vi "Receive Topic Message.vi"(7 "Topic Actor in":refnum<class "Topic Actor.lvclass">, 8 "error in (no error)":errorcluster, 10 "Message in":refnum<class "Message Interface.lvclass">) -> (0 "error out":errorcluster, 3 "Stop?":bool, 5 "Topic Actor out":refnum<class "Topic Actor.lvclass">)   [LabVIEW 2016, in "Stream Mediator.lvlib" / "Topic Actor.lvclass"]
doc: "--\nCopyright © 2017 Composed SystemsI All rights reserved.\n\nAuthor: Jon McBee <jon.mcbee@composed.io>\n\nThis library is provided \"AS IS\" ,WITHOUT WARRANTIES OR\nCONDITIONS OF ANY KIND, either express or implied.\n\nComposed Systems -- composed.io\n\nStream 0.0.1.1\nJon McBee - Composed Systems\nCopyright (c) 2017, Composed Systems"
uses:
  <userlib>/Composed Systems/Stream/Mediator/Classes/Topic Actor/Topic Actor.lvclass
  <userlib>/Composed Systems/Stream/Mediator/Classes/Message Interface/Message Interface.lvclass
  <userlib>/Composed Systems/Stream/Mediator/Classes/Topic Actor Command Interface/Topic Actor Command Interface.lvclass
  <userlib>/Composed Systems/Stream/Mediator/Classes/Topic Actor/Topic Actor.lvclass/Topic Actor.ctl
  <userlib>/Composed Systems/Stream/Mediator/Classes/Message Transport Interface/Message Transport Interface.lvclass
  <userlib>/Composed Systems/Stream/Mediator/Classes/Subscriber Look Up Table/Subscriber Look Up Table.lvclass
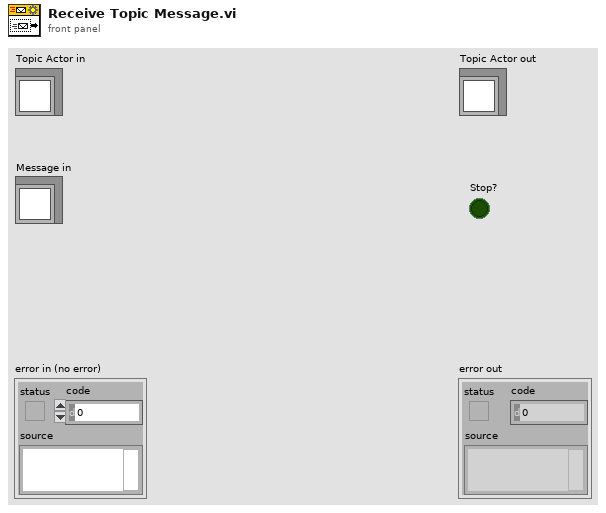
[diagram p1: front panel]
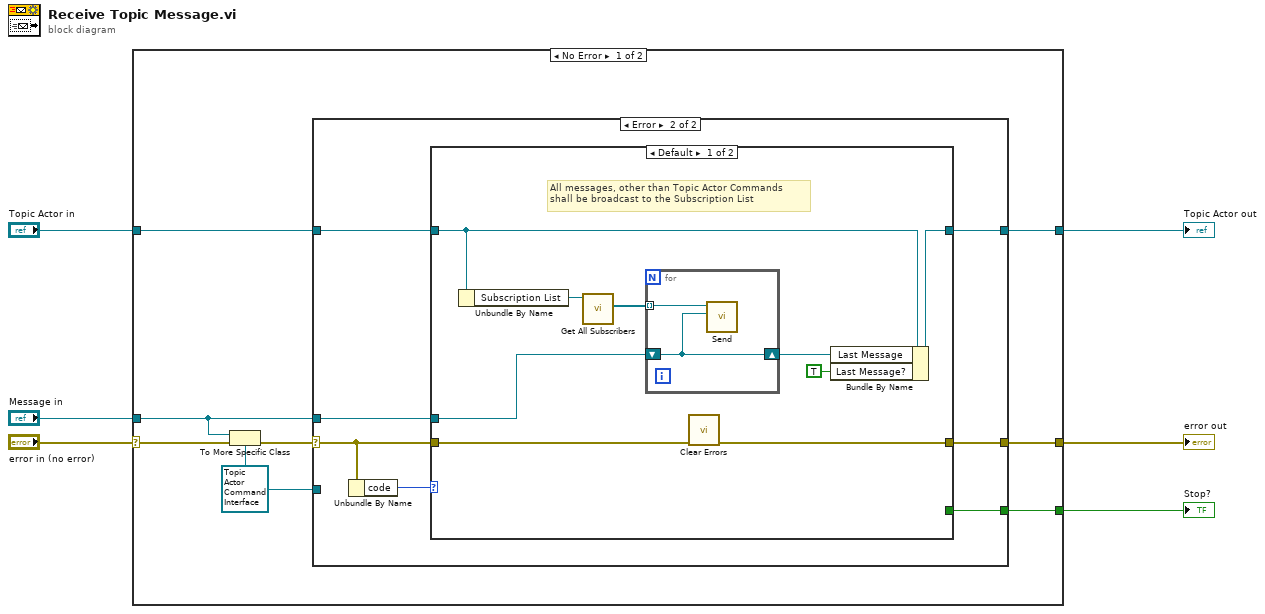
[diagram p0: block diagram]
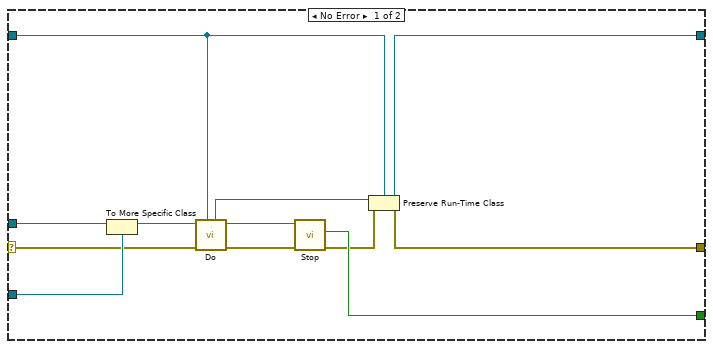
[diagram p2: hidden frame]
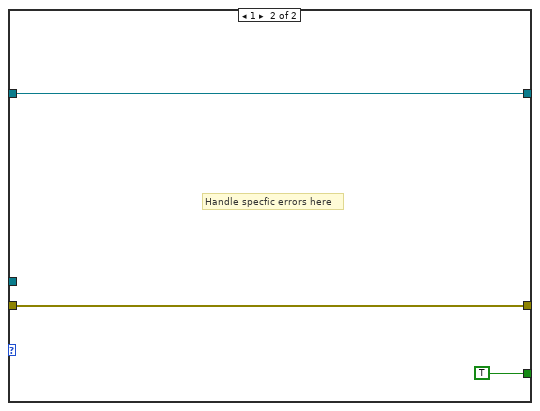
[diagram p3: hidden frame]
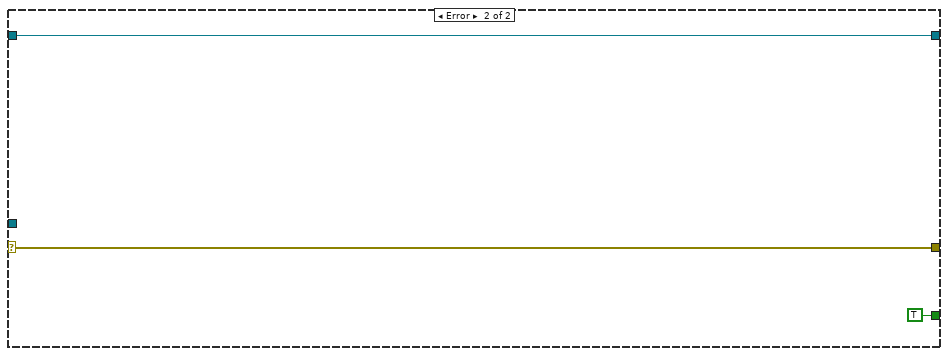
[diagram p4: hidden frame]
diagram:
  n1 = case shown="No Error" "error in (no error)" {
    selector: "error in (no error)" -> [w9 w50]
    tunnel: [w8 w50] -> w5
    tunnel: [w11 w49] -> w3
    tunnel: "Topic Actor in" -> [w12 w49]
    tunnel: "Message in" -> [w10 _]
    tunnel: [w7 TRUE ("Stop?")] -> w1
    frame No Error {
      w13 = refnum<class "Topic Actor Command Interface.lvclass"> refnum ("Topic Actor Command Interface.lvclass")
      n2 = To More Specific Class(target class=w13, reference=w10, error in=w9) -> (error out=w14:errorcluster)  [unwired: 1 out]
      n3 = case shown="Error" w14 {
        selector: w14 -> [w24 w30]
        tunnel: [w18 w32] -> w11
        tunnel: w12 -> [w17 w33]
        tunnel: w10 -> [w26 w28]
        tunnel: w13 -> [w25 _]
        tunnel: [w15 w31] -> w8
        tunnel: [w20 w27] -> w7
        frame No Error {
          n4 = To More Specific Class(target class=w25, reference=w26) -> (specific class reference=w23:refnum<class "Topic Actor Command Interface.lvclass">)  [unwired: 1 in, 1 out]
          n5 = call-dynamic "Do.vi"("Topic Actor in"=w17, "error in (no error)"=w24, "Topic Actor Command in"=w23) -> ("error out"=w21:errorcluster, "Topic Actor Command out"=w22:refnum<class "Topic Actor Command Interface.lvclass">, "Topic Actor out"=w19:refnum<class "Topic Actor.lvclass">)  [unwired: 6 in]
          n6 = call-dynamic "Stop.vi"("error in (no error)"=w21, "Topic Actor Command Interface in"=w22) -> ("error out"=w16:errorcluster, "Stop?"=w20:bool)  [unwired: 7 in, 1 out]
          n7 = Preserve Run-Time Class(object in=w19, error in=w16, 2:w17) -> (object out=w18:refnum<class "Topic Actor.lvclass">, error out=w15:errorcluster)
        }
        frame Error {
          n8 = Unbundle By Name(w30) -> ("code"=w29:i32)
          n9 = case shown="Default" w29 {
            tunnel: [w39 w46] -> w32
            tunnel: w33 -> [w40 w46]
            tunnel: [w34 w47] -> w31
            tunnel: w30 -> [w42 w47]
            tunnel: w28 -> [w41 _]
            tunnel: [_ TRUE] -> w27
            frame Default {
              # "All messages, other than Topic Actor Commands\nshall be broadcast to the Subscription List"
              n10 = Unbundle By Name(w40) -> ("Subscription List"=w36:refnum<class "Subscriber Look Up Table.lvclass">)
              n11 = call <userlib>:"Get All Subscribers.vi"("Subscriber Look Up Table in"=w36) -> ("Subscribers"=w35:refnum<class "Message Transport Interface.lvclass">[])  [unwired: 8 in, 2 out]
              n12 = for {
                shift-right: [w44] -> w38
                shift-left: w41 -> [w44]
                tunnel: w35 -> [w43] mode=indexing
                n13 = call-dynamic "Send.vi"("Message"=w44, "Message Transport Interface in"=w43) -> ()  [unwired: 7 in, 3 out]
              }
              n14 = call <vilib>:"Clear Errors.vi"("error in (no error)"=w42) -> ("error out"=w34:errorcluster)  [unwired: 5 in, 1 out]
              n15 = Bundle By Name(cluster=w40, "Last Message"=w38, "Last Message?"=TRUE) -> (w39:refnum<class "Topic Actor.lvclass">)
            }
            frame 1 {
              # "Handle specfic errors here"
            }
          }
        }
      }
    }
    frame Error {
    }
  }
  "error out" <- w5
  "Topic Actor out" <- w3
  "Stop?" <- w1
